vi "Read Resampler Configuration.vi"(8 "error in (no error)":errorcluster, 11 "Resampler in":refnum<class "Resampler.lvclass">) -> (0 "error out":errorcluster, 2 "Resampler Configuration":T1={"Group"="p", "Reference channel"="", "Channels to resample"=[]}, 3 "Resampler out":refnum<class "Resampler.lvclass">)   [LabVIEW 2024, in "Resampler.lvclass"]
uses:
  Resampler.lvclass
  C:/Nano/fedor2024/labview/LabActor/Template Module/Template Module.lvclass
  Resampler Configuration.ctl
  Template Module/Template Module.lvclass/Template Module.ctl
  Template Module/Read Configuration.vi
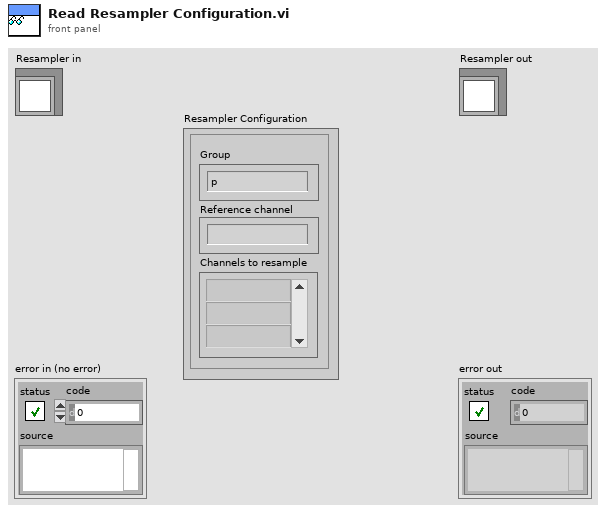
[diagram p1: front panel]
types:
  T1 = typedef "Resampler Configuration.ctl" = cluster{"Group":string, "Reference channel":string, "Channels to resample":string[]}
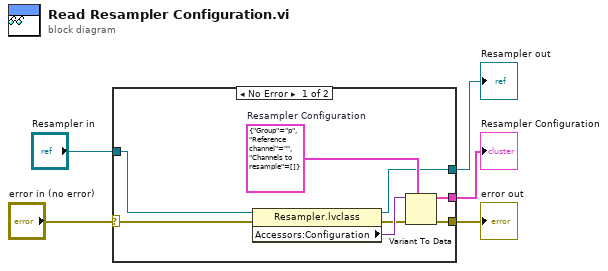
[diagram p0: block diagram]
diagram:
  n1 = case shown="No Error" "error in (no error)" {
    selector: "error in (no error)" -> [w13 w14]
    tunnel: [w9 w14] -> w4
    tunnel: [w7 w15] -> w2
    tunnel: "Resampler in" -> [w6 w15]
    tunnel: [w8 _] -> w1
    frame No Error {
      w10 = T1 {"Group"="p", "Reference channel"="", "Channels to resample"=[]}  # Resampler Configuration
      n2 = property class="Resampler.lvclass"(reference=w6, error in=w13) -> (reference out=w7:refnum<class "Resampler.lvclass">, error out=w11:errorcluster, "Accessors:Configuration"=w12:variant)
      n3 = Variant To Data(error in=w11, type=w10, Variant=w12) -> (data=w8:T1, error out=w9:errorcluster)
    }
    frame Error {
    }
  }
  "error out" <- w4
  "Resampler out" <- w2
  "Resampler Configuration" <- w1
